vi "Read_Joint_States_C.vi"(4 "node":string, 5 "error in":errorcluster, 8 "Units (deg)":enum16{"Radians", "Degrees"}(ring)=enum."Degrees") -> (0 "error out":errorcluster, 1 "right Positions":T1 {"w2" scale=-175.25..175.25; "w1" scale=-90.0..120.0; "w0" scale=-175.25..175.25; "e1" scale=-3.0..150.0; "e0" scale=-173.5..173.5; "s1" scale=-123.0..60.0; "s0" scale=-141.0..51.0}, 2 "left Positions":T1 {"w2" scale=-175.25..175.25; "w1" scale=-90.0..120.0; "w0" scale=-175.25..175.25; "e1" scale=-3.0..150.0; "e0" scale=-173.5..173.5; "s1" scale=-123.0..60.0; "s0" scale=-141.0..51.0}, 3 "Joint States":T2(array[cluster]))   [LabVIEW 2013]
doc: "Read all the current joint states (names, positions, velocity, and efforts)"
uses:
  ROS/Code/JointPositions.ctl
panel:
  out "Reply":string
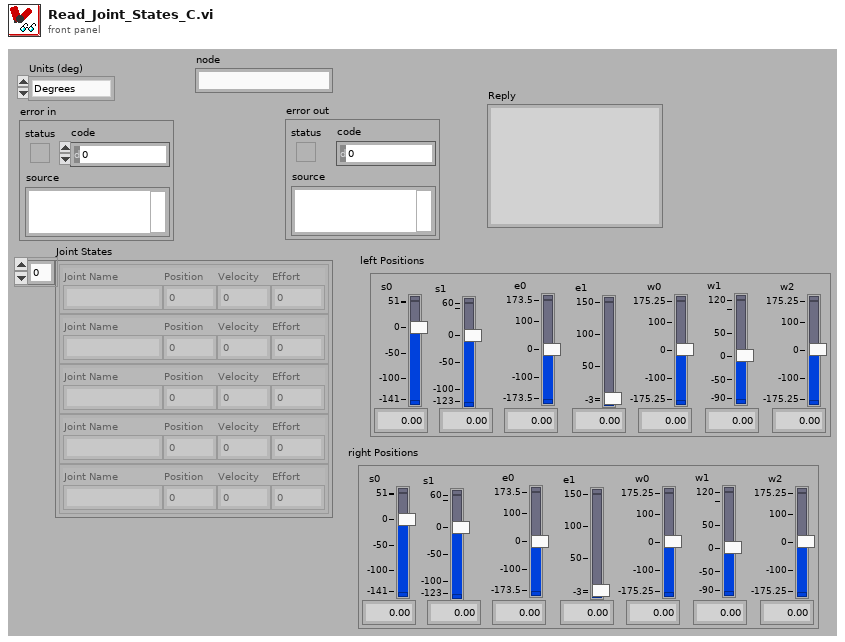
[diagram p1: front panel]
types:
  T1 = typedef "JointPositions.ctl" = cluster{"e0":dbl, "e1":dbl, "s0":dbl, "s1":dbl, "w0":dbl, "w1":dbl, "w2":dbl}
  T2 = cluster{"Joint Name":string, "Position":dbl, "Velocity":dbl, "Effort":dbl}[]
  T3 = typedef "_ROSControl.ctl" = cluster{"topic port":u16, "Node":string, "topic":string, "type":string, "node port":u32, "error ":errorcluster, "Direction":T4, "APIs":string[]}
  T4 = typedef "_ROSDirection.ctl" = enum16{"Node", "Publisher", "Subscriber", "Service Client"}
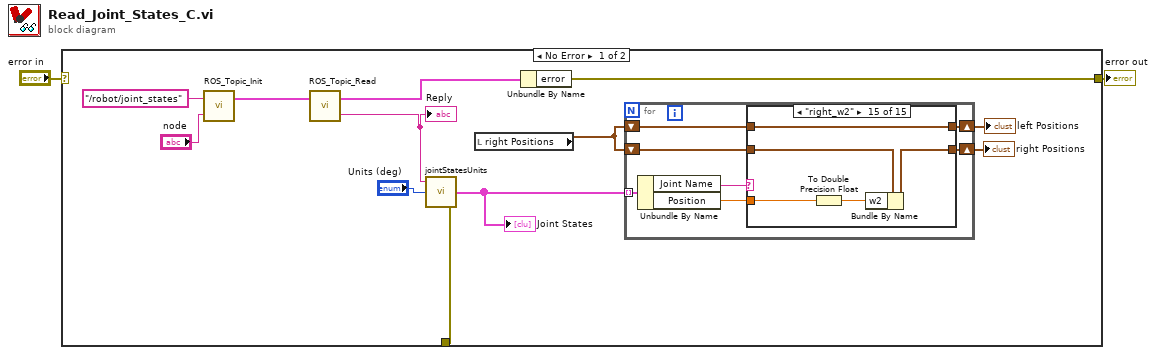
[diagram p0: block diagram]
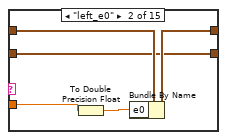
[diagram p3: hidden frame]
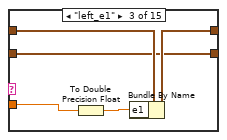
[diagram p4: hidden frame]
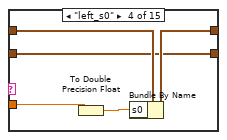
[diagram p5: hidden frame]
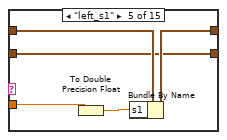
[diagram p6: hidden frame]
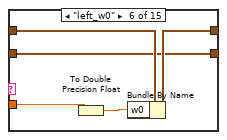
[diagram p7: hidden frame]
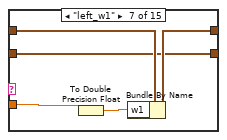
[diagram p8: hidden frame]
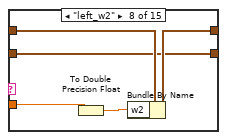
[diagram p9: hidden frame]
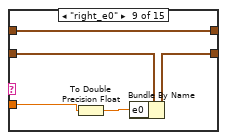
[diagram p10: hidden frame]
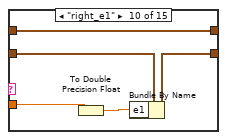
[diagram p11: hidden frame]
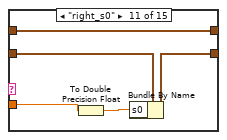
[diagram p12: hidden frame]
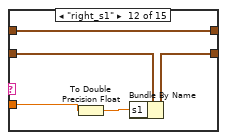
[diagram p13: hidden frame]
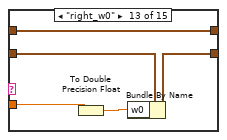
[diagram p14: hidden frame]
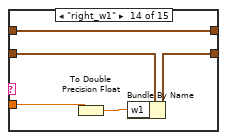
[diagram p15: hidden frame]
diagram:
  n1 = case shown="No Error" "error in" {
    selector: "error in" -> [_ w94]
    tunnel: [w14 w94] -> w2
    tunnel: [w9 _] -> _
    frame No Error {
      n2 = call "ROS_Topic_Init.vi"("node"="node", "topic"="/robot/joint_states") -> ("ROS out"=w11:T3)  [unwired: 1 in]
      n3 = call "ROS_Topic_Read.vi"("ROS in"=w11) -> ("Reply"=w7:string, "ROS out"=w10:T3)  [unwired: 1 in]
      "Reply" <- w7
      n4 = call "jointStatesUnits.vi"("Units (deg)"="Units (deg)", "msg in"=w7) -> ("error out"=w9:errorcluster, "Joint States"=w3:T2)  [unwired: 1 in, 1 out]
      "Joint States" <- w3
      n5 = local read "right Positions"() -> (w4:T1)
      n6 = Unbundle By Name(w10) -> ("error"=w14:errorcluster)
      n7 = for {
        tunnel: w3 -> [w21] mode=indexing
        shift-right: [w20] -> w5
        shift-left: w4 -> [w19]
        shift-right: [w15] -> w6
        shift-left: w4 -> [w16]
        n8 = Unbundle By Name(w21) -> ("Joint Name"=w18:string, "Position"=w17:dbl)
        n9 = case shown="\"right_w2\"" w18 {
          tunnel: [w23 w28 w33 w38 w43 w48 w53 w58 w59 w64 w69 w74 w79 w84 w89] -> w20
          tunnel: w19 -> [w23 w27 w32 w37 w42 w47 w52 w57 w59 w64 w69 w74 w79 w84 w89]
          tunnel: w17 -> [_ w25 w30 w35 w40 w45 w50 w55 w62 w67 w72 w77 w82 w87 w92]
          tunnel: w16 -> [w22 w24 w29 w34 w39 w44 w49 w54 w61 w66 w71 w76 w81 w86 w91]
          tunnel: [w22 w24 w29 w34 w39 w44 w49 w54 w60 w65 w70 w75 w80 w85 w90] -> w15
          frame Default {
          }
          frame "left_e0" {
            n10 = To Double Precision Float(number=w25) -> (double precision float=w26:dbl)
            n11 = Bundle By Name(cluster=w27, "e0"=w26) -> (w28:T1)
          }
          frame "left_e1" {
            n12 = To Double Precision Float(number=w30) -> (double precision float=w31:dbl)
            n13 = Bundle By Name(cluster=w32, "e1"=w31) -> (w33:T1)
          }
          frame "left_s0" {
            n14 = To Double Precision Float(number=w35) -> (double precision float=w36:dbl)
            n15 = Bundle By Name(cluster=w37, "s0"=w36) -> (w38:T1)
          }
          frame "left_s1" {
            n16 = To Double Precision Float(number=w40) -> (double precision float=w41:dbl)
            n17 = Bundle By Name(cluster=w42, "s1"=w41) -> (w43:T1)
          }
          frame "left_w0" {
            n18 = To Double Precision Float(number=w45) -> (double precision float=w46:dbl)
            n19 = Bundle By Name(cluster=w47, "w0"=w46) -> (w48:T1)
          }
          frame "left_w1" {
            n20 = To Double Precision Float(number=w50) -> (double precision float=w51:dbl)
            n21 = Bundle By Name(cluster=w52, "w1"=w51) -> (w53:T1)
          }
          frame "left_w2" {
            n22 = To Double Precision Float(number=w55) -> (double precision float=w56:dbl)
            n23 = Bundle By Name(cluster=w57, "w2"=w56) -> (w58:T1)
          }
          frame "right_e0" {
            n24 = To Double Precision Float(number=w62) -> (double precision float=w63:dbl)
            n25 = Bundle By Name(cluster=w61, "e0"=w63) -> (w60:T1)
          }
          frame "right_e1" {
            n26 = To Double Precision Float(number=w67) -> (double precision float=w68:dbl)
            n27 = Bundle By Name(cluster=w66, "e1"=w68) -> (w65:T1)
          }
          frame "right_s0" {
            n28 = To Double Precision Float(number=w72) -> (double precision float=w73:dbl)
            n29 = Bundle By Name(cluster=w71, "s0"=w73) -> (w70:T1)
          }
          frame "right_s1" {
            n30 = To Double Precision Float(number=w77) -> (double precision float=w78:dbl)
            n31 = Bundle By Name(cluster=w76, "s1"=w78) -> (w75:T1)
          }
          frame "right_w0" {
            n32 = To Double Precision Float(number=w82) -> (double precision float=w83:dbl)
            n33 = Bundle By Name(cluster=w81, "w0"=w83) -> (w80:T1)
          }
          frame "right_w1" {
            n34 = To Double Precision Float(number=w87) -> (double precision float=w88:dbl)
            n35 = Bundle By Name(cluster=w86, "w1"=w88) -> (w85:T1)
          }
          frame "right_w2" {
            n36 = To Double Precision Float(number=w92) -> (double precision float=w93:dbl)
            n37 = Bundle By Name(cluster=w91, "w2"=w93) -> (w90:T1)
          }
        }
      }
      "right Positions" <- w6
      "left Positions" <- w5
    }
    frame Error {
    }
  }
  "error out" <- w2
